vi "Action Worker.vi"(7 "Name (\"\" to Use UUID)":string) -> ()   [LabVIEW 2017, in "Action Worker Mode Example.lvlib"]
doc: "------------- lvcsm -------------\n[CSMStates]\nItem 0 = \"Idle\"\nItem 1 = \"CSM Documentation\"\nItem 2 = \"VI Reference\"\nItem 3 = \"Error Handler\"\nItem 4 = \"Critical Error\"\nItem 5 = \"Target Timeout Error\"\nItem 6 = \"Target Error\"\nItem 7 = \"Initialize Core Data\"\nItem 8 = \"Async Response\"\nItem 9 = \"Response\"\nItem 10 = \"Async Message Posted\"\nItem 11 = \"Exit\"\nItem 12 = \"Data: Initialize\"\nItem 13 = \"Data: Update Indicators\"\nItem 14 = \"Data: Cleanup\"\nItem 15 = \"Macro: Initialize\"\nItem 16 = \"Macro: Exit\"\nItem 17 = \"API: API1\"\nItem 18 = \"API: API2\"\nItem 19 = \"DoSth: DoA\"\nItem 20 = \"DoSth: Error\"\n\n[CSMStatus]\nItem 0 = \"Error Occurred@Error Handler\""
uses:
  Action Worker Mode Example.lvlib
  user.lib/_NEVSTOP/Communicable State Machine(CSM)/AdvanceAPI/CSM - Make String Arguments Safe.vi
  user.lib/_NEVSTOP/Communicable State Machine(CSM)/AdvanceAPI/CSM - Break Down Multiple States String.vi
  user.lib/_NEVSTOP/Communicable State Machine(CSM)/AdvanceAPI/CSM - Compact Multiple States.vi
  user.lib/_NEVSTOP/Communicable State Machine(CSM)/AdvanceAPI/CSM - Keywords.vi
  user.lib/_NEVSTOP/Communicable State Machine(CSM)/Communicable State Machine.lvlib
panel:
  out "Error Occurred":errorcluster
  out "State History":string
  # "#CSM-Example Overview\n\nDemonstrates the Worker Mode in the CSM framework. In Worker Mode, multiple clonable CSM instances operate as sub-modules. To avoid naming conflicts, CSM automatically appends a “#” postfix to worker module names. When a message is sent to worker, the first idle instance handles it using a fair queue mechanism. From the outside, the system behaves as if only one module is running, while all CSM concepts—such as synchronous, asynchronous, and status messages—remain unchanged.\n\nIn this example, four worker instances of worker run in the background. Check the history log to see which instance processed each message."
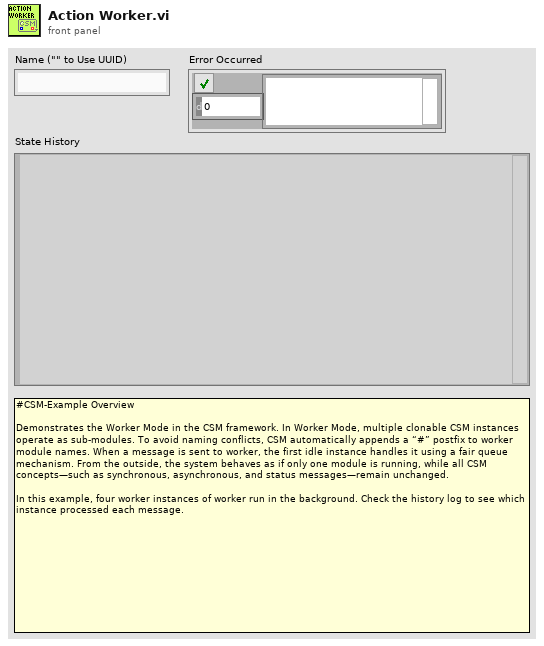
[diagram p1: front panel]
types:
  T1 = enum32{"Invalid", "Standard", "Closed", "Hidden", "Minimized", "Maximized"}
  T2 = enum32{"invalid app kind", "Development System", "Run Time System", "Student Edition", "Embedded LabVIEW", "Evaluation", "Custom"}
  T3 = typedef "Communicable State Machine.lvlib/_CSM_Response Source Message.ctl" = cluster{"‘State":string, "’Arguments":string, "’Error":errorcluster}
  T4 = cluster{"Current VI Reference":refnum<vi>, "Close Panel on Exit?":bool}
  T5 = cluster{"Core":cluster{"Current VI Reference":refnum<vi>, "Close Panel on Exit?":bool}, "Your Boolean data":bool, "Your string data":string}
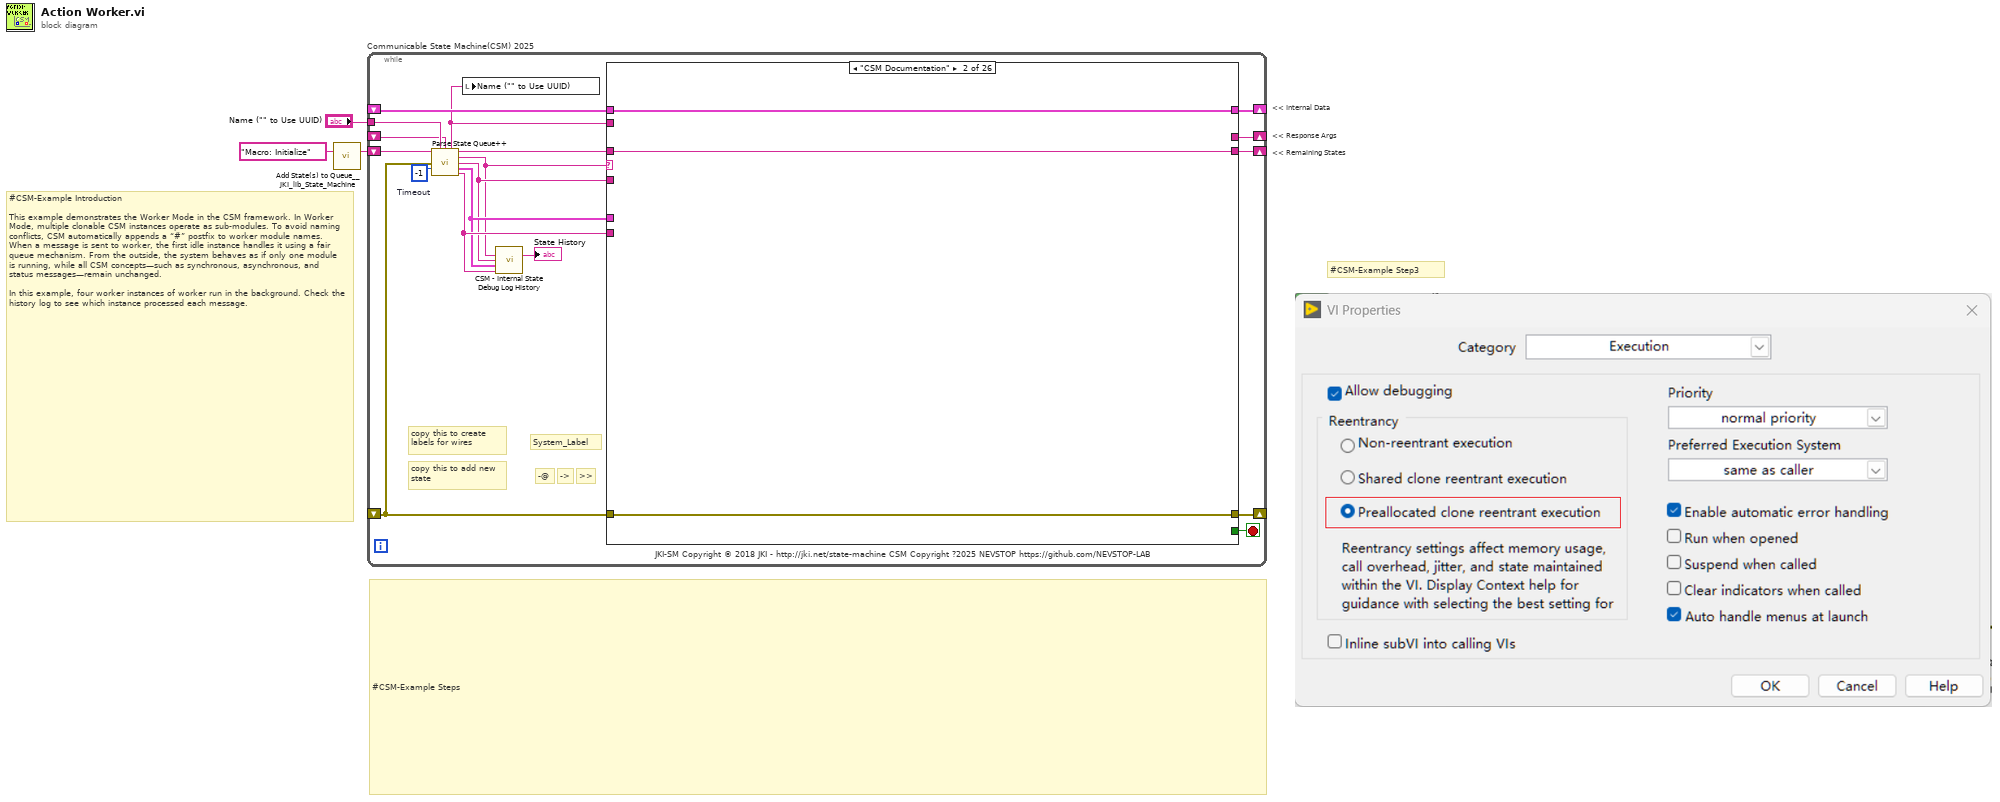
[diagram p0: block diagram]
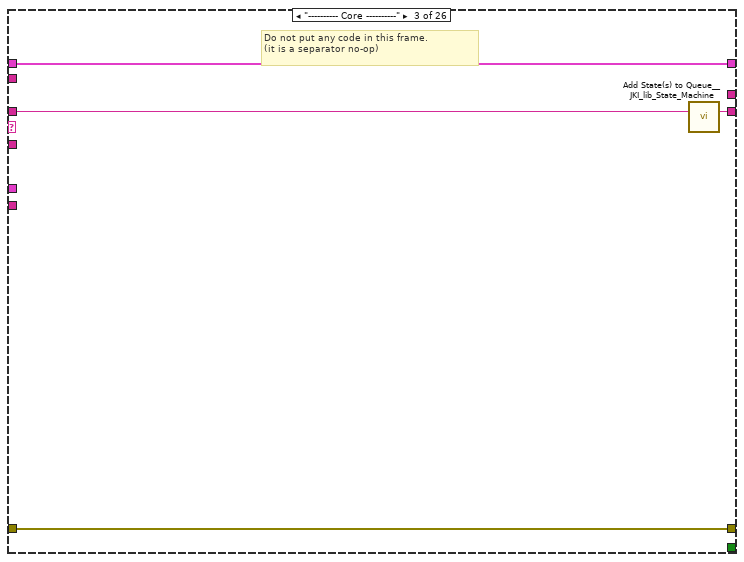
[diagram p3: hidden frame]
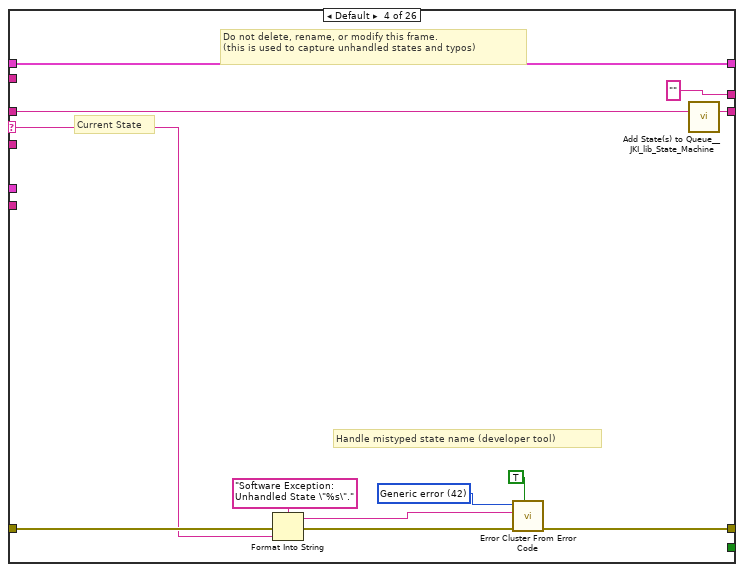
[diagram p4: hidden frame]
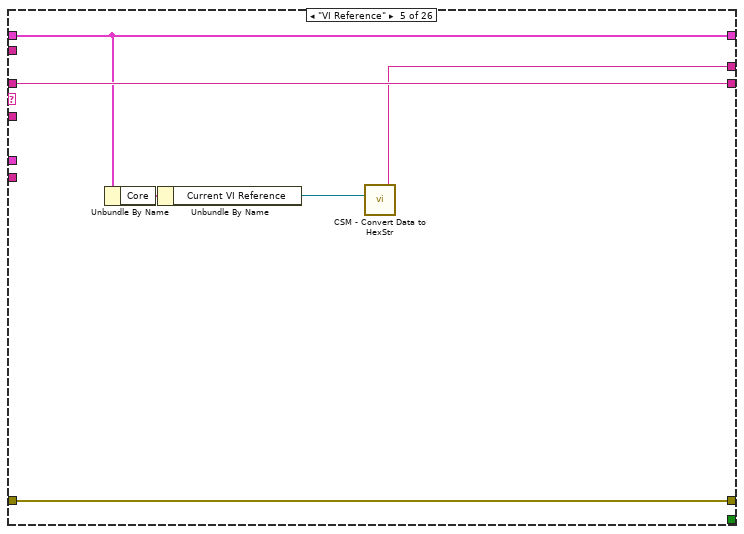
[diagram p5: hidden frame]
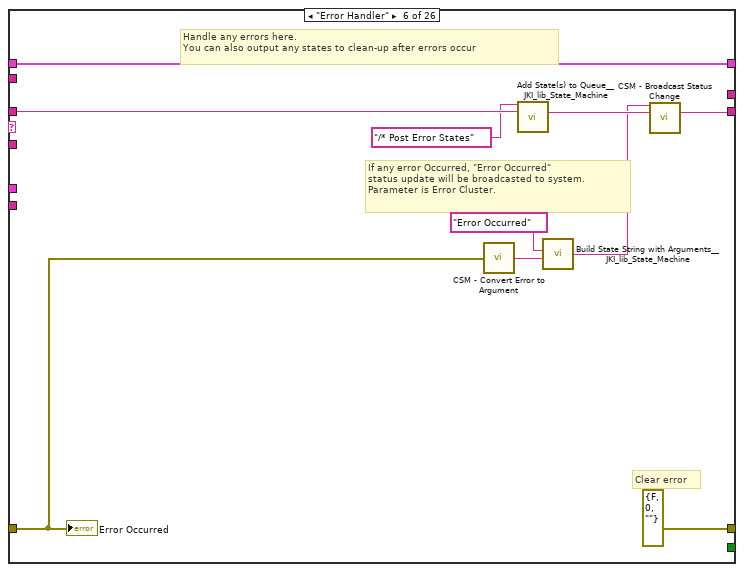
[diagram p6: hidden frame]
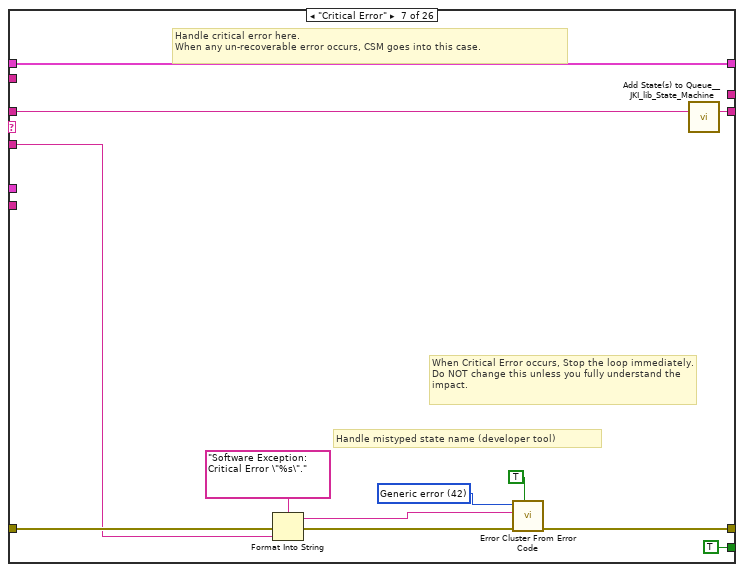
[diagram p7: hidden frame]
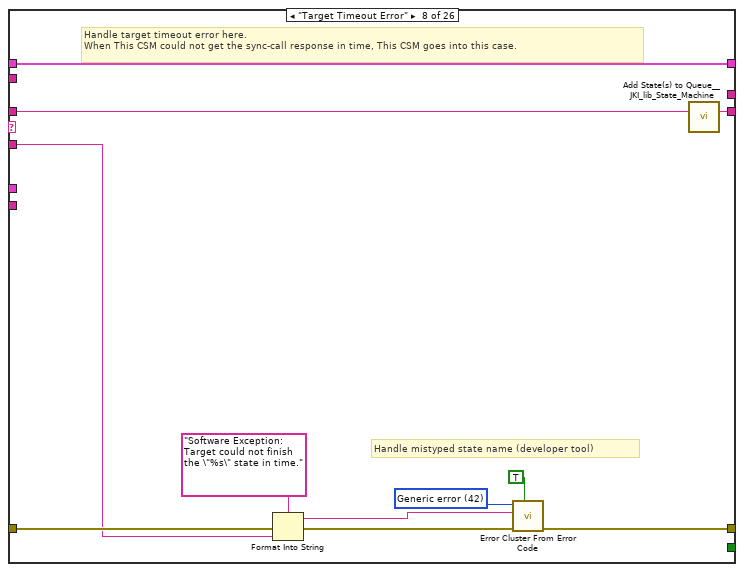
[diagram p8: hidden frame]
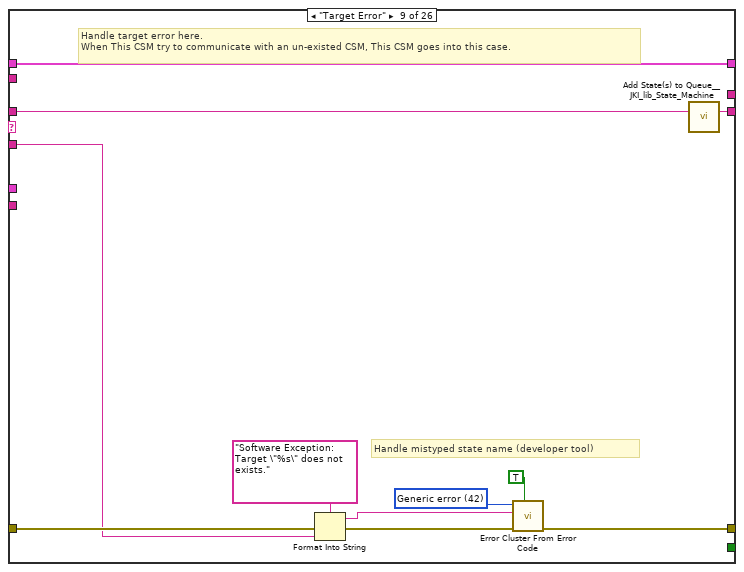
[diagram p9: hidden frame]
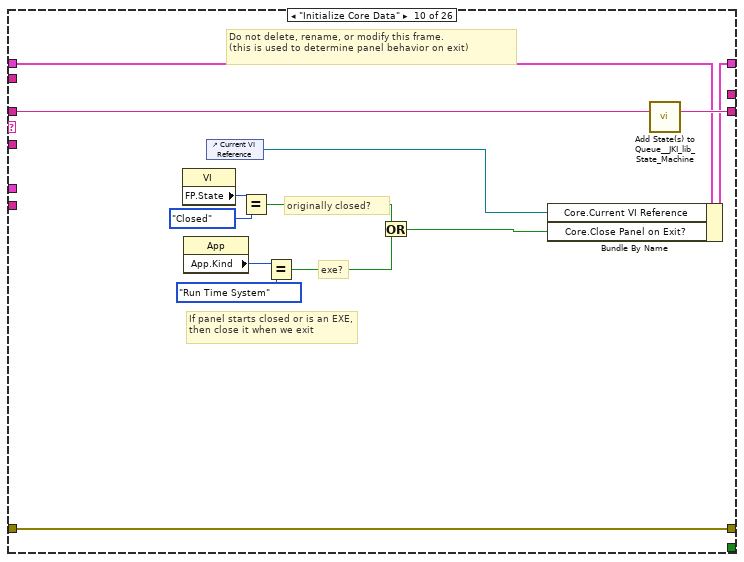
[diagram p10: hidden frame]
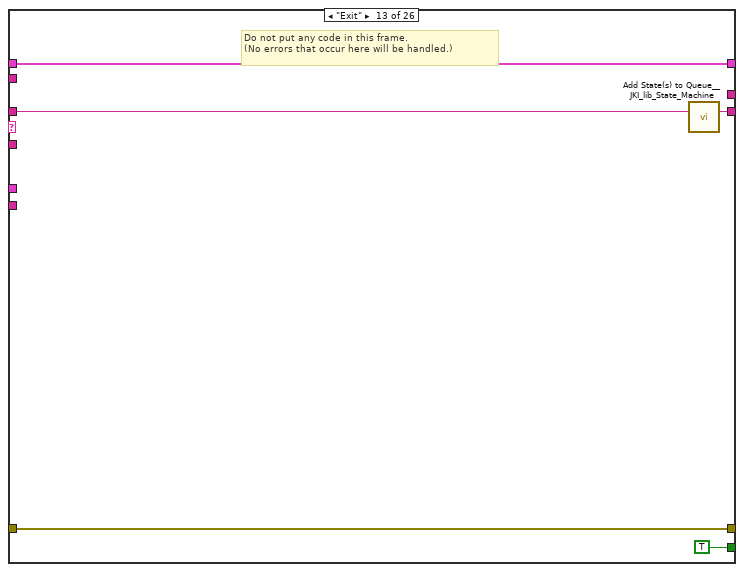
[diagram p13: hidden frame]
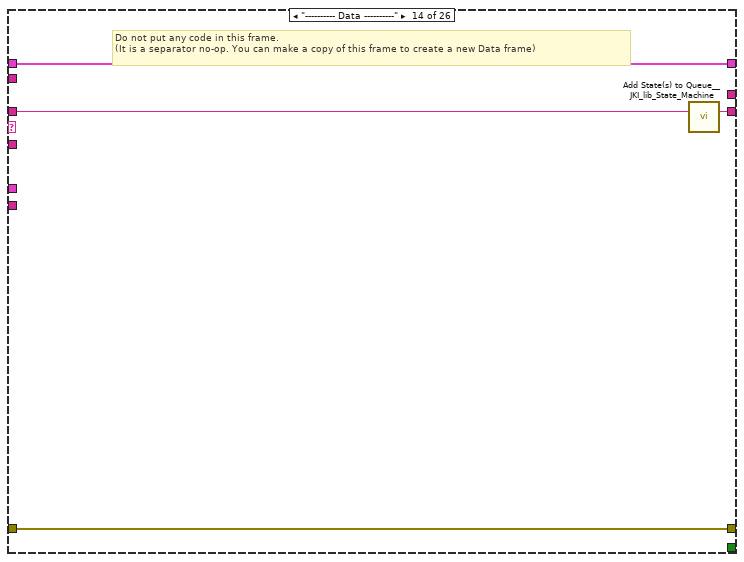
[diagram p14: hidden frame]
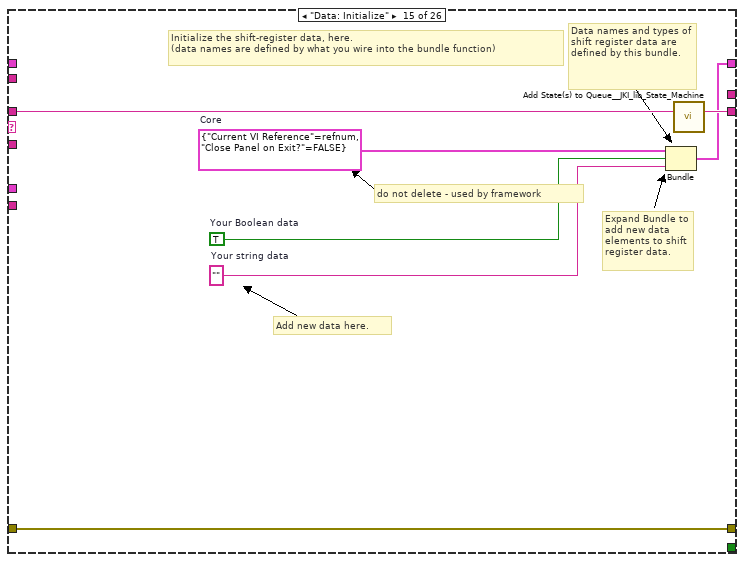
[diagram p15: hidden frame]
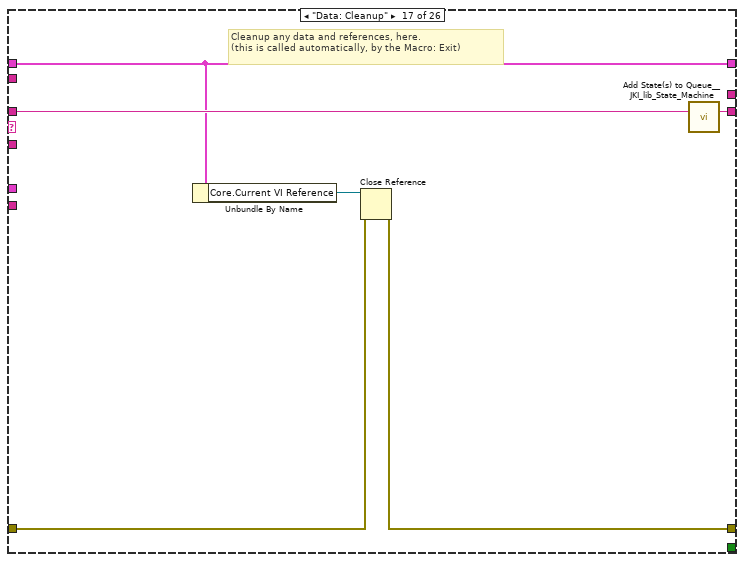
[diagram p17: hidden frame]
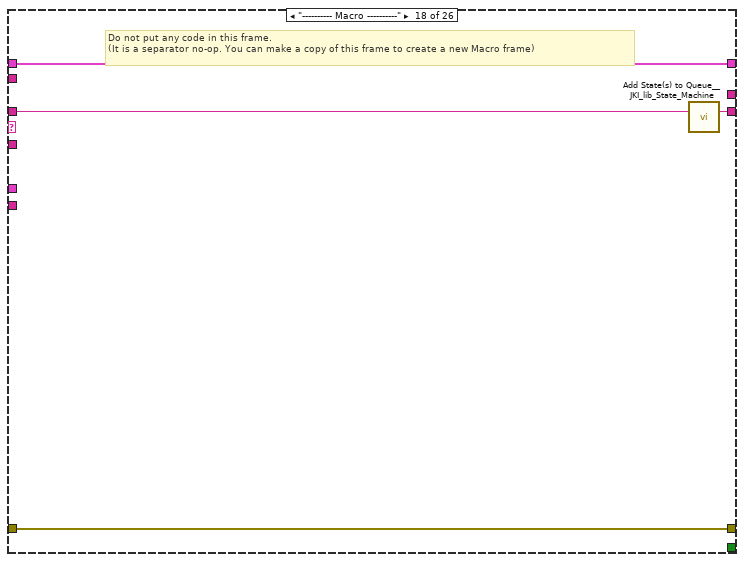
[diagram p18: hidden frame]
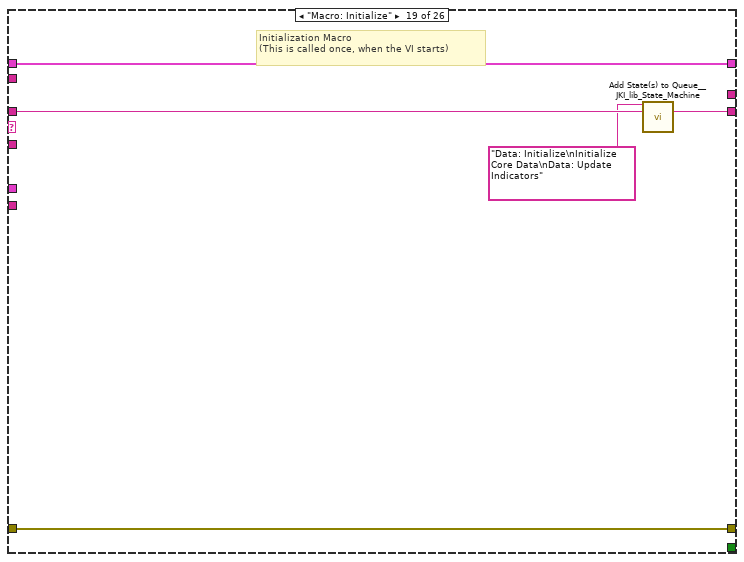
[diagram p19: hidden frame]
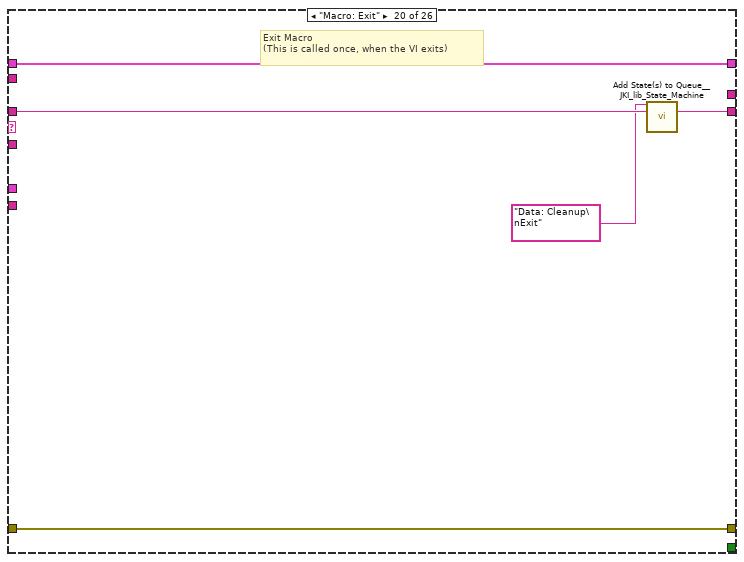
[diagram p20: hidden frame]
diagram:
  # "#CSM-Example Step3"
  # "#CSM-Example Steps"
  # "#CSM-Example Introduction\n\nThis example demonstrates the Worker Mode in the CSM framework. In Worker Mode, multiple clonable CSM instances operate as sub-modules. To avoid naming conflicts, CSM automatically appends a “#” postfix to worker module names. When a message is sent to worker, the first idle instance handles it using a fair queue mechanism. From the outside, the system behaves as if only one module is running, while all CSM concepts—such as synchronous, asynchronous, and status messages—remain unchanged.\n\nIn this example, four worker instances of worker run in the background. Check the history log to see which instance processed each message."
  # "<< Internal Data"
  # "<< Response Args"
  # "<< Remaining States"
  n1 = call <vilib>:"Add State(s) to Queue__JKI_lib_State_Machine.vi"("State(s) in (\"\")"="Macro: Initialize") -> ("States Out"=w1:string)  [unwired: 14 in]
  n2 = while "Communicable State Machine(CSM) 2025" {
    shift-right: [w16] -> _
    shift-left: _ -> [w15]
    shift-right: [w19] -> _
    shift-left: _ -> [w14]
    shift-right: [w18] -> _
    shift-left: w1 -> [w20]
    tunnel: "Name (\"\" to Use UUID)" -> [w11]
    shift-right: [w12] -> _
    shift-left: _ -> [w6]
    stop <- w17 stop-if-true
    w13 = -1  # Timeout
    # "JKI-SM Copyright © 2018 JKI - http://jki.net/state-machine CSM Copyright ?2025 NEVSTOP https://github.com/NEVSTOP-LAB"
    # ">>"
    # "copy this to add new state"
    # "->"
    # "-@"
    # "copy this to create labels for wires"
    # "System_Label"
    n3 = call "Parse State Queue++.vi"("State Queue"=w20, "Name (\"\" to Use UUID)"=w11, "Response Arguments"=w6, "Previous Error"=w14, "Dequeue (1 ms)"=w13) -> ("Name Used"=w5:string, "Remaining States"=w21:string, "Current State"=w7:string, "Arguments"=w8:string, ">> Response Source Message >>"=w9:T3, ">> Source CSM >>"=w10:string)  [unwired: 5 in]
    n4 = local write "Name (\"\" to Use UUID)"(w5) -> ()
    n5 = call "CSM - Internal State Debug Log History.vi"("State"=w7, "Arguments (\"\")"=w8, ">> Response Source Message >>"=w9, "Source (\"\")"=w10) -> ("Debug Log"=→"State History":string)  [unwired: 11 in]
    n6 = case shown="\"CSM Documentation\"" w7 {
      selector: w7 -> [_ _ _ w33 _ _ _ _ _ _ _ _ _ _ _ _ _ _ _ _ _ _ _ _ _ _]
      tunnel: w21 -> [w22 w26 w31 w37 w48 w59 w65 w76 w87 w106 w108 w111 w117 w121 w128 w130 w137 w141 w146 w151 w153 w157 w162 w169 w174 w179]
      tunnel: w8 -> [_ _ _ _ _ _ w61 w72 w83 _ _ _ _ _ _ _ _ _ _ _ _ _ w160 _ _ _]
      tunnel: w15 -> [w23 w25 w28 w35 w47 w57 w63 w74 w85 w99 w107 w110 w115 w118 _ w129 w132 w138 w143 w148 w152 w156 w161 w166 w171 w177]
      tunnel: [w24 w27 w29 w39 w49 errorcluster {"status"=FALSE, "code"=0, "source"=""} ("error out") w67 w78 w89 w103 w109 w112 w114 w119 w125 w131 w133 w139 w144 w149 w154 w158 w163 w167 w172 errorcluster {"status"=TRUE, "code"=12345, "source"="This is a simulated error"} ("error out")] -> w19
      tunnel: w14 -> [w24 w27 w29 w38 w49 w50 w66 w77 w88 w103 w109 w112 w114 w119 w125 w131 w134 w139 w144 w149 w154 w158 w163 w167 w172 _]
      tunnel: [w22 w26 w30 w36 w48 w52 w64 w75 w86 w105 w108 w111 w116 w120 w127 w130 w136 w140 w145 w150 w153 w157 w162 w168 w173 w178] -> w18
      tunnel: [_ _ _ _ _ _ TRUE _ _ _ _ _ TRUE _ _ _ _ _ _ _ _ _ _ _ _ _] -> w17
      tunnel: [w23 w25 w28 w35 w47 w57 w63 w74 w85 w104 w107 w110 w115 w118 w126 w129 w132 w138 w143 w148 w152 w156 w161 w166 w171 w177] -> w16
      tunnel: w10 -> [_ _ _ _ _ _ _ _ _ _ _ _ _ _ _ _ _ _ _ _ _ _ _ _ _ _]
      tunnel: w9 -> [_ _ _ _ _ _ _ _ _ _ _ _ _ _ _ _ _ _ _ _ _ _ _ _ _ _]
      tunnel: [_ _ _ "" w44 _ _ _ _ _ _ _ _ _ _ _ _ _ _ _ _ "API1 Response" w159 _ "DoA Finished" "Error!!"] -> w12
      tunnel: w5 -> [_ _ _ _ _ _ _ _ _ _ _ _ _ _ _ _ _ _ _ _ _ _ _ _ _ _]
      frame "", "Idle" {
        # "README FIRST\n \nThis VI template should be used by dragging & dropping it from the Functions palette onto the Block Diagram of a new, blank VI, which will place it's contents into the blank VI. \nDo not edit the VI found in the palette.  Only edit the state machine after it is placed into your blank VI.\n \nFor instructions on how to use the JKI State Machine, examples and video tutorials, visit: http://jki.net/state-machine/\n\nJKI State Machine™\nhttp://jki.net/state-machine/\nCopyright (C) 2005-2018, JKI <info@jki.net>\nALL RIGHTS RESERVED\n\nFor information about CSM, visit: https://github.com/NEVSTOP-LAB"
        # "executes when the state queue is empty"
      }
      frame "CSM Documentation" {
      }
      frame "---------- Core ----------" {
        # "Do not put any code in this frame.\n(it is a separator no-op)"
        n7 = call <vilib>:"Add State(s) to Queue__JKI_lib_State_Machine.vi"("State(s) in (\"\")"=w31) -> ("States Out"=w30:string)  [unwired: 14 in]
      }
      frame Default {
        w42 = 42 items=["No error", "Argument error", "Memory is full", "Out of zone", "End of file", "File already open", "Generic file I/O error", "File not found", "File permission error", "Disk is full", "Duplicate path", "Too many files open", "System feature not enabled", "Resource file not found", "Cannot add resource", "Resource not found", "Image not found", "Image memory error", "Pen does not exist", "Config type invalid", "Config token not found", "Config parse error", "Config memory error", "Bad external code format", "Bad external code offset", "External code not present", "Null window", "Destroy window error", "Null menu", "Print aborted", "Bad print record", "Print driver error", "Windows error during printing", "Memory error during printing", "Print dialog error", "Generic print error", "Invalid device refnum", "Device not found", "Device parameter error", "Device unit error", "Cannot open device", "Device call aborted", "Generic error", "Cancelled by user", "Object ID too low", "Object ID too high", "Object not in heap", "Unknown heap", "Unknown object (invalid DefProc)", "Unknown object (DefProc not in table)", "Message out of range", "Invalid (null) method", "Unknown message", "Manager call not supported", "Bad address", "Network operation in progress", "Network operation timed out", "Connection is busy", "Network attribute not supported", "Network error", "Address in use", "System out of memory", "Connection aborted", "Connection refused", "Not connected", "Already connected", "Connection closed", "Initialization error (interapplication manager)", "Bad occurrence", "Wait on unbound occurrence handler", "Occurrence queue overflow", "Datalog type conflict", "Unused", "Unrecognized type (interapplication manager)", "Memory corrupt", "Failed to make temporary DLL", "Old CIN version", "Drag socket not found", "Failed to load drop-object", "Failed to register OLE object", "Failed to release OLE object", "Format specifier type mismatch", "Unknown format specifier", "Too few format specifiers", "Too many format specifiers", "Scan failed", "Newer CIN version", "Error converting to variant", "Runtime menu error", "Password tampered", "Variant attribute not found", "Incompatible variant data type", "Event data is not available", "Event Store is not present", "Occurrence is not found", "Event Queue is not created", "Event info is not available", "Refnum passed is NULL", "Error retrieving Class GUID", "Error retrieving CoClass GUID", "Error retrieving TypeLib GUID.", "Bad built application magic bytes.", "Specific driver is different from the specific driver associated with the Logical Name.", "There is no session opened to the class driver.", "Max Error", "MAX - Error with config objects", "MAX - Error loading configuration", "MAX - Group not supported"]
        # "Current State"
        # "Do not delete, rename, or modify this frame.\n(this is used to capture unhandled states and typos)"
        # "Handle mistyped state name (developer tool)"
        n8 = Format Into String(format string="Software Exception: Unhandled State \"%s\"." ("message"), error in=w38, w33) -> (resulting string=w41:string, error out=w40:errorcluster)  [unwired: 1 in]
        n9 = call <vilib>:"Error Cluster From Error Code.vi"("show call chain? (False)"=TRUE, "error in (no error)"=w40, "error message (\"\")"=w41, "error code (0)"=w42) -> ("error out"=w39:errorcluster)  [unwired: 5 in]
        n10 = call <vilib>:"Add State(s) to Queue__JKI_lib_State_Machine.vi"("State(s) in (\"\")"=w37) -> ("States Out"=w36:string)  [unwired: 14 in]
      }
      frame "VI Reference" {
        n11 = Unbundle By Name(w47) -> ("Core"=w46:T4)
        n12 = Unbundle By Name(w46) -> ("Current VI Reference"=w45:refnum<vi>)
        n13 = call "CSM - Convert Data to HexStr.vi"("Variant"=w45) -> ("HEX String (0-9,A-F)"=w44:string)  [unwired: 8 in]
      }
      frame "Error Handler" {
        # "If any error Occurred, \"Error Occurred\" \nstatus update will be broadcasted to system.\nParameter is Error Cluster."
        # "Handle any errors here.\nYou can also output any states to clean-up after errors occur"
        # "Clear error"
        n14 = call "CSM - Convert Error to Argument.vi"("Error"=w50) -> ("Argument"=w54:string)  [unwired: 4 in]
        n15 = call <vilib>:"Add State(s) to Queue__JKI_lib_State_Machine.vi"("State(s) in Front (\"\")"="/* Post Error States", "State(s) in (\"\")"=w59) -> ("States Out"=w53:string)  [unwired: 13 in]
        n16 = call <vilib>:"Build State String with Arguments__JKI_lib_State_Machine.vi"("Arguments (\"\")"=w54, "State"="Error Occurred" ("Status with Arguments")) -> ("State with Arguments"=w51:string)  [unwired: 4 in]
        n17 = call "CSM - Broadcast Status Change.vi"("Status With Arguments"=w51, "State Queue"=w53) -> ("Remaining States"=w52:string)  [unwired: 13 in]
        "Error Occurred" <- w50
      }
      frame "Critical Error" {
        w70 = 42 items=["No error", "Argument error", "Memory is full", "Out of zone", "End of file", "File already open", "Generic file I/O error", "File not found", "File permission error", "Disk is full", "Duplicate path", "Too many files open", "System feature not enabled", "Resource file not found", "Cannot add resource", "Resource not found", "Image not found", "Image memory error", "Pen does not exist", "Config type invalid", "Config token not found", "Config parse error", "Config memory error", "Bad external code format", "Bad external code offset", "External code not present", "Null window", "Destroy window error", "Null menu", "Print aborted", "Bad print record", "Print driver error", "Windows error during printing", "Memory error during printing", "Print dialog error", "Generic print error", "Invalid device refnum", "Device not found", "Device parameter error", "Device unit error", "Cannot open device", "Device call aborted", "Generic error", "Cancelled by user", "Object ID too low", "Object ID too high", "Object not in heap", "Unknown heap", "Unknown object (invalid DefProc)", "Unknown object (DefProc not in table)", "Message out of range", "Invalid (null) method", "Unknown message", "Manager call not supported", "Bad address", "Network operation in progress", "Network operation timed out", "Connection is busy", "Network attribute not supported", "Network error", "Address in use", "System out of memory", "Connection aborted", "Connection refused", "Not connected", "Already connected", "Connection closed", "Initialization error (interapplication manager)", "Bad occurrence", "Wait on unbound occurrence handler", "Occurrence queue overflow", "Datalog type conflict", "Unused", "Unrecognized type (interapplication manager)", "Memory corrupt", "Failed to make temporary DLL", "Old CIN version", "Drag socket not found", "Failed to load drop-object", "Failed to register OLE object", "Failed to release OLE object", "Format specifier type mismatch", "Unknown format specifier", "Too few format specifiers", "Too many format specifiers", "Scan failed", "Newer CIN version", "Error converting to variant", "Runtime menu error", "Password tampered", "Variant attribute not found", "Incompatible variant data type", "Event data is not available", "Event Store is not present", "Occurrence is not found", "Event Queue is not created", "Event info is not available", "Refnum passed is NULL", "Error retrieving Class GUID", "Error retrieving CoClass GUID", "Error retrieving TypeLib GUID.", "Bad built application magic bytes.", "Specific driver is different from the specific driver associated with the Logical Name.", "There is no session opened to the class driver.", "Max Error", "MAX - Error with config objects", "MAX - Error loading configuration", "MAX - Group not supported"]
        # "Handle critical error here.\nWhen any un-recoverable error occurs, CSM goes into this case."
        # "When Critical Error occurs, Stop the loop immediately. Do NOT change this unless you fully understand the impact."
        # "Handle mistyped state name (developer tool)"
        n18 = Format Into String(format string="Software Exception: Critical Error \"%s\"." ("message"), error in=w66, w61) -> (resulting string=w69:string, error out=w68:errorcluster)  [unwired: 1 in]
        n19 = call <vilib>:"Error Cluster From Error Code.vi"("show call chain? (False)"=TRUE, "error in (no error)"=w68, "error message (\"\")"=w69, "error code (0)"=w70) -> ("error out"=w67:errorcluster)  [unwired: 5 in]
        n20 = call <vilib>:"Add State(s) to Queue__JKI_lib_State_Machine.vi"("State(s) in (\"\")"=w65) -> ("States Out"=w64:string)  [unwired: 14 in]
      }
      frame "Target Timeout Error" {
        w81 = 42 items=["No error", "Argument error", "Memory is full", "Out of zone", "End of file", "File already open", "Generic file I/O error", "File not found", "File permission error", "Disk is full", "Duplicate path", "Too many files open", "System feature not enabled", "Resource file not found", "Cannot add resource", "Resource not found", "Image not found", "Image memory error", "Pen does not exist", "Config type invalid", "Config token not found", "Config parse error", "Config memory error", "Bad external code format", "Bad external code offset", "External code not present", "Null window", "Destroy window error", "Null menu", "Print aborted", "Bad print record", "Print driver error", "Windows error during printing", "Memory error during printing", "Print dialog error", "Generic print error", "Invalid device refnum", "Device not found", "Device parameter error", "Device unit error", "Cannot open device", "Device call aborted", "Generic error", "Cancelled by user", "Object ID too low", "Object ID too high", "Object not in heap", "Unknown heap", "Unknown object (invalid DefProc)", "Unknown object (DefProc not in table)", "Message out of range", "Invalid (null) method", "Unknown message", "Manager call not supported", "Bad address", "Network operation in progress", "Network operation timed out", "Connection is busy", "Network attribute not supported", "Network error", "Address in use", "System out of memory", "Connection aborted", "Connection refused", "Not connected", "Already connected", "Connection closed", "Initialization error (interapplication manager)", "Bad occurrence", "Wait on unbound occurrence handler", "Occurrence queue overflow", "Datalog type conflict", "Unused", "Unrecognized type (interapplication manager)", "Memory corrupt", "Failed to make temporary DLL", "Old CIN version", "Drag socket not found", "Failed to load drop-object", "Failed to register OLE object", "Failed to release OLE object", "Format specifier type mismatch", "Unknown format specifier", "Too few format specifiers", "Too many format specifiers", "Scan failed", "Newer CIN version", "Error converting to variant", "Runtime menu error", "Password tampered", "Variant attribute not found", "Incompatible variant data type", "Event data is not available", "Event Store is not present", "Occurrence is not found", "Event Queue is not created", "Event info is not available", "Refnum passed is NULL", "Error retrieving Class GUID", "Error retrieving CoClass GUID", "Error retrieving TypeLib GUID.", "Bad built application magic bytes.", "Specific driver is different from the specific driver associated with the Logical Name.", "There is no session opened to the class driver.", "Max Error", "MAX - Error with config objects", "MAX - Error loading configuration", "MAX - Group not supported"]
        # "Handle target timeout error here.\nWhen This CSM could not get the sync-call response in time, This CSM goes into this case."
        # "Handle mistyped state name (developer tool)"
        n21 = Format Into String(format string="Software Exception: Target could not finish the \"%s\" state in time." ("message"), error in=w77, w72) -> (resulting string=w80:string, error out=w79:errorcluster)  [unwired: 1 in]
        n22 = call <vilib>:"Error Cluster From Error Code.vi"("show call chain? (False)"=TRUE, "error in (no error)"=w79, "error message (\"\")"=w80, "error code (0)"=w81) -> ("error out"=w78:errorcluster)  [unwired: 5 in]
        n23 = call <vilib>:"Add State(s) to Queue__JKI_lib_State_Machine.vi"("State(s) in (\"\")"=w76) -> ("States Out"=w75:string)  [unwired: 14 in]
      }
      frame "Target Error" {
        w92 = 42 items=["No error", "Argument error", "Memory is full", "Out of zone", "End of file", "File already open", "Generic file I/O error", "File not found", "File permission error", "Disk is full", "Duplicate path", "Too many files open", "System feature not enabled", "Resource file not found", "Cannot add resource", "Resource not found", "Image not found", "Image memory error", "Pen does not exist", "Config type invalid", "Config token not found", "Config parse error", "Config memory error", "Bad external code format", "Bad external code offset", "External code not present", "Null window", "Destroy window error", "Null menu", "Print aborted", "Bad print record", "Print driver error", "Windows error during printing", "Memory error during printing", "Print dialog error", "Generic print error", "Invalid device refnum", "Device not found", "Device parameter error", "Device unit error", "Cannot open device", "Device call aborted", "Generic error", "Cancelled by user", "Object ID too low", "Object ID too high", "Object not in heap", "Unknown heap", "Unknown object (invalid DefProc)", "Unknown object (DefProc not in table)", "Message out of range", "Invalid (null) method", "Unknown message", "Manager call not supported", "Bad address", "Network operation in progress", "Network operation timed out", "Connection is busy", "Network attribute not supported", "Network error", "Address in use", "System out of memory", "Connection aborted", "Connection refused", "Not connected", "Already connected", "Connection closed", "Initialization error (interapplication manager)", "Bad occurrence", "Wait on unbound occurrence handler", "Occurrence queue overflow", "Datalog type conflict", "Unused", "Unrecognized type (interapplication manager)", "Memory corrupt", "Failed to make temporary DLL", "Old CIN version", "Drag socket not found", "Failed to load drop-object", "Failed to register OLE object", "Failed to release OLE object", "Format specifier type mismatch", "Unknown format specifier", "Too few format specifiers", "Too many format specifiers", "Scan failed", "Newer CIN version", "Error converting to variant", "Runtime menu error", "Password tampered", "Variant attribute not found", "Incompatible variant data type", "Event data is not available", "Event Store is not present", "Occurrence is not found", "Event Queue is not created", "Event info is not available", "Refnum passed is NULL", "Error retrieving Class GUID", "Error retrieving CoClass GUID", "Error retrieving TypeLib GUID.", "Bad built application magic bytes.", "Specific driver is different from the specific driver associated with the Logical Name.", "There is no session opened to the class driver.", "Max Error", "MAX - Error with config objects", "MAX - Error loading configuration", "MAX - Group not supported"]
        # "Handle target error here.\nWhen This CSM try to communicate with an un-existed CSM, This CSM goes into this case."
        # "Handle mistyped state name (developer tool)"
        n24 = Format Into String(format string="Software Exception: Target \"%s\" does not exists." ("message"), error in=w88, w83) -> (resulting string=w91:string, error out=w90:errorcluster)  [unwired: 1 in]
        n25 = call <vilib>:"Error Cluster From Error Code.vi"("show call chain? (False)"=TRUE, "error in (no error)"=w90, "error message (\"\")"=w91, "error code (0)"=w92) -> ("error out"=w89:errorcluster)  [unwired: 5 in]
        n26 = call <vilib>:"Add State(s) to Queue__JKI_lib_State_Machine.vi"("State(s) in (\"\")"=w87) -> ("States Out"=w86:string)  [unwired: 14 in]
      }
      frame "Initialize Core Data" {
        # "Do not delete, rename, or modify this frame.\n(this is used to determine panel behavior on exit)"
        # "originally closed?"
        # "exe?"
        # "If panel starts closed or is an EXE, then close it when we exit"
        n27 = property class="VI"() -> ("FP.State"=w96:T1)  [unwired: 2 in, 2 out]
        n28 = property class="App"() -> ("App.Kind"=w102:T2)  [unwired: 2 in, 2 out]
        n29 = control-ref of="Current VI Reference"() -> (w97:refnum<vi>)
        n30 = Equal?(x=w96, y=T1."Closed" ("Front Panel Window:State")) -> (x = y?=w94:bool)
        n31 = Equal?(x=w102, y=T2."Run Time System" ("Application:Kind")) -> (x = y?=w100:bool)
        n32 = Or(x=w94, y=w100) -> (x .or. y?=w98:bool)
        n33 = Bundle By Name(cluster=w99, "Core.Current VI Reference"=w97, "Core.Close Panel on Exit?"=w98) -> (w104:T5)
        n34 = call <vilib>:"Add State(s) to Queue__JKI_lib_State_Machine.vi"("State(s) in (\"\")"=w106) -> ("States Out"=w105:string)  [unwired: 14 in]
      }
      frame "Async Response", "Response" {
      }
      frame "Async Message Posted" {
      }
      frame "Exit" {
        # "Do not put any code in this frame.\n(No errors that occur here will be handled.)"
        n35 = call <vilib>:"Add State(s) to Queue__JKI_lib_State_Machine.vi"("State(s) in (\"\")"=w117) -> ("States Out"=w116:string)  [unwired: 14 in]
      }
      frame "---------- Data ----------" {
        # "Do not put any code in this frame.\n(It is a separator no-op. You can make a copy of this frame to create a new Data frame)"
        n36 = call <vilib>:"Add State(s) to Queue__JKI_lib_State_Machine.vi"("State(s) in (\"\")"=w121) -> ("States Out"=w120:string)  [unwired: 14 in]
      }
      frame "Data: Initialize" {
        w122 = T4 {"Current VI Reference"=refnum, "Close Panel on Exit?"=FALSE}  # Core
        w124 = TRUE  # Your Boolean data
        w123 = ""  # Your string data
        # "do not delete - used by framework"
        # "Expand Bundle to add new data elements to shift register data."
        # "Add new data here."
        # "Data names and types of shift register data are defined by this bundle."
        # "Initialize the shift-register data, here.\n(data names are defined by what you wire into the bundle function)"
        n37 = Bundle("Core"=w122, "Your Boolean data"=w124, "Your string data"=w123) -> (w126:T5)  [unwired: 1 in]
        n38 = call <vilib>:"Add State(s) to Queue__JKI_lib_State_Machine.vi"("State(s) in (\"\")"=w128) -> ("States Out"=w127:string)  [unwired: 14 in]
      }
      frame "Data: Update Indicators" {
      }
      frame "Data: Cleanup" {
        # "Cleanup any data and references, here.\n(this is called automatically, by the Macro: Exit)"
        n39 = Unbundle By Name(w132) -> ("Core.Current VI Reference"=w135:refnum<vi>)
        n40 = Close Reference(reference=w135, error in (no error)=w134) -> (error out=w133:errorcluster)
        n41 = call <vilib>:"Add State(s) to Queue__JKI_lib_State_Machine.vi"("State(s) in (\"\")"=w137) -> ("States Out"=w136:string)  [unwired: 14 in]
      }
      frame "---------- Macro ----------" {
        # "Do not put any code in this frame.\n(It is a separator no-op. You can make a copy of this frame to create a new Macro frame)"
        n42 = call <vilib>:"Add State(s) to Queue__JKI_lib_State_Machine.vi"("State(s) in (\"\")"=w141) -> ("States Out"=w140:string)  [unwired: 14 in]
      }
      frame "Macro: Initialize" {
        # "Initialization Macro\n(This is called once, when the VI starts)"
        n43 = call <vilib>:"Add State(s) to Queue__JKI_lib_State_Machine.vi"("State(s) in Front (\"\")"="Data: Initialize\nInitialize Core Data\nData: Update Indicators", "State(s) in (\"\")"=w146) -> ("States Out"=w145:string)  [unwired: 13 in]
      }
      frame "Macro: Exit" {
        # "Exit Macro\n(This is called once, when the VI exits)"
        n44 = call <vilib>:"Add State(s) to Queue__JKI_lib_State_Machine.vi"("State(s) in Front (\"\")"="Data: Cleanup\nExit", "State(s) in (\"\")"=w151) -> ("States Out"=w150:string)  [unwired: 13 in]
      }
      frame "---------- API ----------" {
        # "Do not put any code in this frame.\n(It is a separator no-op. This category is recommended to use for external API)"
      }
      frame "API: API1" {
        # "If you need to tell who triggered this state , use this string. If it's this case itself, this string is \"\"."
        # "Deal with the parameter if any"
        # "Connect this to return the response of your API"
        # "Copy/Rename this case for your own API"
      }
      frame "API: API2" {
        # "unpack HexStr  to Variant\nif complex parameter is needed."
        # "Copy/Rename this case for your own API"
        n45 = call "CSM - Convert HexStr to Data.vi"("HEX String"=w160) -> ()  [unwired: 7 in, 2 out]
        n46 = disable-structure shown="Disabled" {
          disable-tunnel: [w164 "API2 Response"] -> w159
          frame Disabled {
            # "pack variant to hexstr \nif complex response is needed."
            # "complex Response"
            n47 = call "CSM - Convert Data to HexStr.vi"() -> ("HEX String (0-9,A-F)"=w164:string)  [unwired: 9 in]
          }
          frame Enabled {
          }
        }
      }
      frame "---------- DoSth ----------" {
        # "Template Separator\n(You can make a copy of, or modify, this frame)"
        n48 = call <vilib>:"Add State(s) to Queue__JKI_lib_State_Machine.vi"("State(s) in (\"\")"=w169) -> ("States Out"=w168:string)  [unwired: 14 in]
      }
      frame "DoSth: DoA" {
        # "#CSM-Example Step1"
        n49 = call <vilib>:"Add State(s) to Queue__JKI_lib_State_Machine.vi"("State(s) in (\"\")"=w174) -> ("States Out"=w173:string)  [unwired: 14 in]
      }
      frame "DoSth: Error" {
        # "#CSM-Example Step2"
        n50 = call <vilib>:"Add State(s) to Queue__JKI_lib_State_Machine.vi"("State(s) in (\"\")"=w179) -> ("States Out"=w178:string)  [unwired: 14 in]
      }
    }
  }
